vi "Write Tags.vi"(8 "error in (no error)":errorcluster, 11 "State in":T1={"State"=enum."Idle", "Start Time"=timestamp(0 s since 1904-01-01), "Configuration"={"Cycle Period"=0.0, "Ismatech"={"VISA resource name"="", "Simulated?"=FALSE, "Pump Number"=1.0, "Reverse?"=FALSE}, "Masterflex"={"VISA resource name"="", "Simulated?"=FALSE, "Pump Number"=1.0, "Reverse?"=FALSE}, "Mettler"={"VISA resource name"="", "Simulated?"=FALSE}, "Bronkhorst M13 Flow Meter"={"VISA resource name"="", "Simulated?"=FALSE, "Smoothing Steps"=1}, "PID 2 Parameters"={"Input Device"=enum."Bronkhorst M13", "Output Device"=enum."Ismatec ISM 831C", "Setpoint"=0.0, "PID gains"={"proportional gain (Kc)"=1.0, "integral time (Ti, min)"=0.01, "derivative time (Td, min)"=0.0}}, "Manual Entry"=0.0, "Auto?"=TRUE, "PID range"={"PID High"=100.0, "PID Low"=0.0, "High Warning"=100.0}, "Tacmina Settings"={"Analog DAQ Task"="", "Digital DAQ Task"=""}, "KNF SIMDOS Settings"={"VISA resource name"="", "Simulated?"=TRUE}, "ASIA Pump C"={"ASIA Pump #"=0, "channel"=0, "Simulated"=FALSE}, "VICI Settings"={"VISA resource name"="", "Pump ID"="", "Pump Head Vol"=0.0, "Reverse?"=FALSE, "Simulated?"=FALSE}, "FLOM Settings"={"VISA resource name"="", "Simulated?"=TRUE, "Pump Number"=0.0}, "SSI PR/LD Settings"={"VISA resource name"="", "Simulated?"=FALSE}, "Masterflex 75211 Settings"={"Analog DAQ Task"="", "Digital DAQ Task"=""}, "SSI P40 Settings"={"VISA resource name"="", "Simulated?"=TRUE}, "Ismatech 3 Channel Settings"={"VISA resource name"="", "Pump Number"=1, "Channel Number"=0, "Simulated?"=TRUE, "Reverse?"=FALSE}, "Bronkhorst M14 Settings"={"VISA resource name"="", "Simulated?"=FALSE, "Smoothing Steps"=1}, "Reset Totalizer"=FALSE, "Input Num Alarm Settings"=[], "Control Type"=enum."g/min", "Front End Display Options"={"Temperature"=TRUE, "Scale Grams"=FALSE, "Density"=TRUE, "Flow (g/min)"=FALSE, "Flow (ml/min)"=TRUE, "PSIG"=TRUE, "Total Grams"=TRUE, "Updated"=TRUE}}, "Current Time"=timestamp(0 s since 1904-01-01), "PID 1 Parameters"={"Setpoint"=0.0, "PID gains"={"proportional gain (Kc)"=1.0, "integral time (Ti, min)"=0.01, "derivative time (Td, min)"=0.0}}, "First Iteration"=FALSE, "Data"={"Flowmeter (g/min)"=0.0, "Flowmeter (ml/min)"=0.0, "Density"=0.0, "FL Temp"=0.0, "Scale Output (g)"=0.0, "Scale Rate of Change (g/min)"=0.0, "PID 1 Output"=0.0, "PID 2 Process Variable"=0.0, "PID 2 output"=0.0, "Pump Flow"=0.0, "Pump Pressure"=0.0, "Totalized Value"=0.0}, "Process Name"="", "Pump On?"=enum."Off", "Input Error"=FALSE, "Output Error"=FALSE, "Log Started"=FALSE, "PID Overshoot"=FALSE, "Current Setpoint"=0.0} {"PID 1 Parameters"."PID gains"."derivative time (Td, min)" format="%.3f"; "PID 1 Parameters"."PID gains"."integral time (Ti, min)" format="%.3f"; "PID 1 Parameters"."PID gains"."proportional gain (Kc)" format="%.3f"; "Configuration"."Bronkhorst M14 Settings"."Smoothing Steps" min=1 step=1; "Configuration"."Ismatech 3 Channel Settings"."Channel Number" min=0 max=3; "Configuration"."Ismatech 3 Channel Settings"."Pump Number" min=1; "Configuration"."PID range"."PID Low" min=0.0 max=100.0 format="%.2f"; "Configuration"."PID range"."PID High" format="%.2f"; "Configuration"."PID 2 Parameters"."PID gains"."derivative time (Td, min)" format="%.3f"; "Configuration"."PID 2 Parameters"."PID gains"."integral time (Ti, min)" format="%.3f"; "Configuration"."PID 2 Parameters"."PID gains"."proportional gain (Kc)" format="%.3f"; "Configuration"."Bronkhorst M13 Flow Meter"."Smoothing Steps" min=1 step=1; "Configuration"."ASIA Pump C"."channel" min=0 max=1 step=1; "Configuration"."Ismatech"."Pump Number" min=1.0 max=20.0 step=1.0; "Configuration"."Masterflex"."Pump Number" min=1.0 max=20.0 step=1.0}) -> (0 "error out":errorcluster, 3 "State out":T1={"State"=enum."Idle", "Start Time"=timestamp(0 s since 1904-01-01), "Configuration"={"Cycle Period"=0.0, "Ismatech"={"VISA resource name"="", "Simulated?"=FALSE, "Pump Number"=1.0, "Reverse?"=FALSE}, "Masterflex"={"VISA resource name"="", "Simulated?"=FALSE, "Pump Number"=1.0, "Reverse?"=FALSE}, "Mettler"={"VISA resource name"="", "Simulated?"=FALSE}, "Bronkhorst M13 Flow Meter"={"VISA resource name"="", "Simulated?"=FALSE, "Smoothing Steps"=1}, "PID 2 Parameters"={"Input Device"=enum."Bronkhorst M13", "Output Device"=enum."Ismatec ISM 831C", "Setpoint"=0.0, "PID gains"={"proportional gain (Kc)"=1.0, "integral time (Ti, min)"=0.01, "derivative time (Td, min)"=0.0}}, "Manual Entry"=0.0, "Auto?"=TRUE, "PID range"={"PID High"=100.0, "PID Low"=0.0, "High Warning"=100.0}, "Tacmina Settings"={"Analog DAQ Task"="", "Digital DAQ Task"=""}, "KNF SIMDOS Settings"={"VISA resource name"="", "Simulated?"=TRUE}, "ASIA Pump C"={"ASIA Pump #"=0, "channel"=0, "Simulated"=FALSE}, "VICI Settings"={"VISA resource name"="", "Pump ID"="", "Pump Head Vol"=0.0, "Reverse?"=FALSE, "Simulated?"=FALSE}, "FLOM Settings"={"VISA resource name"="", "Simulated?"=TRUE, "Pump Number"=0.0}, "SSI PR/LD Settings"={"VISA resource name"="", "Simulated?"=FALSE}, "Masterflex 75211 Settings"={"Analog DAQ Task"="", "Digital DAQ Task"=""}, "SSI P40 Settings"={"VISA resource name"="", "Simulated?"=TRUE}, "Ismatech 3 Channel Settings"={"VISA resource name"="", "Pump Number"=1, "Channel Number"=0, "Simulated?"=TRUE, "Reverse?"=FALSE}, "Bronkhorst M14 Settings"={"VISA resource name"="", "Simulated?"=FALSE, "Smoothing Steps"=1}, "Reset Totalizer"=FALSE, "Input Num Alarm Settings"=[], "Control Type"=enum."g/min", "Front End Display Options"={"Temperature"=TRUE, "Scale Grams"=FALSE, "Density"=TRUE, "Flow (g/min)"=FALSE, "Flow (ml/min)"=TRUE, "PSIG"=TRUE, "Total Grams"=TRUE, "Updated"=TRUE}}, "Current Time"=timestamp(0 s since 1904-01-01), "PID 1 Parameters"={"Setpoint"=0.0, "PID gains"={"proportional gain (Kc)"=1.0, "integral time (Ti, min)"=0.01, "derivative time (Td, min)"=0.0}}, "First Iteration"=FALSE, "Data"={"Flowmeter (g/min)"=0.0, "Flowmeter (ml/min)"=0.0, "Density"=0.0, "FL Temp"=0.0, "Scale Output (g)"=0.0, "Scale Rate of Change (g/min)"=0.0, "PID 1 Output"=0.0, "PID 2 Process Variable"=0.0, "PID 2 output"=0.0, "Pump Flow"=0.0, "Pump Pressure"=0.0, "Totalized Value"=0.0}, "Process Name"="", "Pump On?"=enum."Off", "Input Error"=FALSE, "Output Error"=FALSE, "Log Started"=FALSE, "PID Overshoot"=FALSE, "Current Setpoint"=0.0} {"PID 1 Parameters"."PID gains"."derivative time (Td, min)" format="%.3f"; "PID 1 Parameters"."PID gains"."integral time (Ti, min)" format="%.3f"; "PID 1 Parameters"."PID gains"."proportional gain (Kc)" format="%.3f"; "Configuration"."Bronkhorst M14 Settings"."Smoothing Steps" min=1 step=1; "Configuration"."Ismatech 3 Channel Settings"."Channel Number" min=0 max=3; "Configuration"."Ismatech 3 Channel Settings"."Pump Number" min=1; "Configuration"."PID range"."PID Low" min=0.0 max=100.0 format="%.2f"; "Configuration"."PID range"."PID High" format="%.2f"; "Configuration"."PID 2 Parameters"."PID gains"."derivative time (Td, min)" format="%.3f"; "Configuration"."PID 2 Parameters"."PID gains"."integral time (Ti, min)" format="%.3f"; "Configuration"."PID 2 Parameters"."PID gains"."proportional gain (Kc)" format="%.3f"; "Configuration"."Bronkhorst M13 Flow Meter"."Smoothing Steps" min=1 step=1; "Configuration"."ASIA Pump C"."channel" min=0 max=1 step=1; "Configuration"."Ismatech"."Pump Number" min=1.0 max=20.0 step=1.0; "Configuration"."Masterflex"."Pump Number" min=1.0 max=20.0 step=1.0})   [LabVIEW 2018, in "Feed Module.lvlib" / "Feed Module Engine.lvlib"]
uses:
  Feed Module Engine.lvlib
  State Cluster.ctl
  State Enum.ctl
  Feed Module/Controls/Feed Module Settings Cluster.ctl
  Ismatec ISM 831C/Controls/Ismatech ISM831C Settings Cluster.ctl
  Masterflex 7550-30/Controls/Settings Cluster.ctl
  Mettler Toledo/Controls/Settings Cluster.ctl
  Bronkhorst M13 Flow Meter/Settings Cluster.ctl
  PID 2 Parameters Cluster.ctl
  PID Input Enum.ctl
  PID 2 Output Enum.ctl
  Tacmina QI/Tacmina QI DAQ Setting.ctl
  KNF Pump/Settings Cluster plus SIMDOS.ctl
  ASIA Pump/Pump Settings.ctl
  VICI M50 Party Mode/Settings Cluster.ctl
  FLOM Pump/Settings Cluster.ctl
  SSI PR Class/SSI PR or LD Settings Cluster.ctl
  Masterflex 75211/Masterflex 75211 DAQ Setting.ctl
  SSI PR Class/SSI P40 Settings Cluster.ctl
  Ismatec 78001/Ismatec 4083.ctl
  Bronkhorst M14 Flow Meter/Settings Cluster.ctl
  Tag VIs/Numeric Alarm Settings Cluster.ctl
  PID 1 Parameters Cluster.ctl
  Tag VIs/Tag FGV Operation Enum.ctl
  Shared Variables/Dynamic Shared Variables.lvlib
  Feed Module/Feed Module.lvlib
  Ismatec ISM 831C/Ismatec ISM 831C.lvlib
  Masterflex 7550-30/Masterflex 7550-30.lvlib
  Mettler Toledo/Mettler Toledo.lvlib
  Bronkhorst M13 Flow Meter/Bronkhorst M13 Flow Meter.lvlib
  Tacmina QI/Tacmina QI.lvlib
  KNF Pump/KNF SIMDOS.lvlib
  ASIA Pump.lvlib
  VICI M50 Party Mode/VICI M6 M50 Party Mode.lvlib
  FLOM Pump/FLOM Pump.lvlib
  SSI PR Class/SSI PR or LD Pump.lvlib
  Masterflex 75211/Masterflex 75211.lvlib
  SSI PR Class/SSI P40 Pump.lvlib
  Ismatec 78001/Ismatec 4308.lvlib
  Bronkhorst M14 Flow Meter/Bronkhorst M14 Flow Meter.lvlib
panel:
  # "Output Instruments"
  # "Input Instruments"
  # "Output Instruments"
  # "Input Instruments"
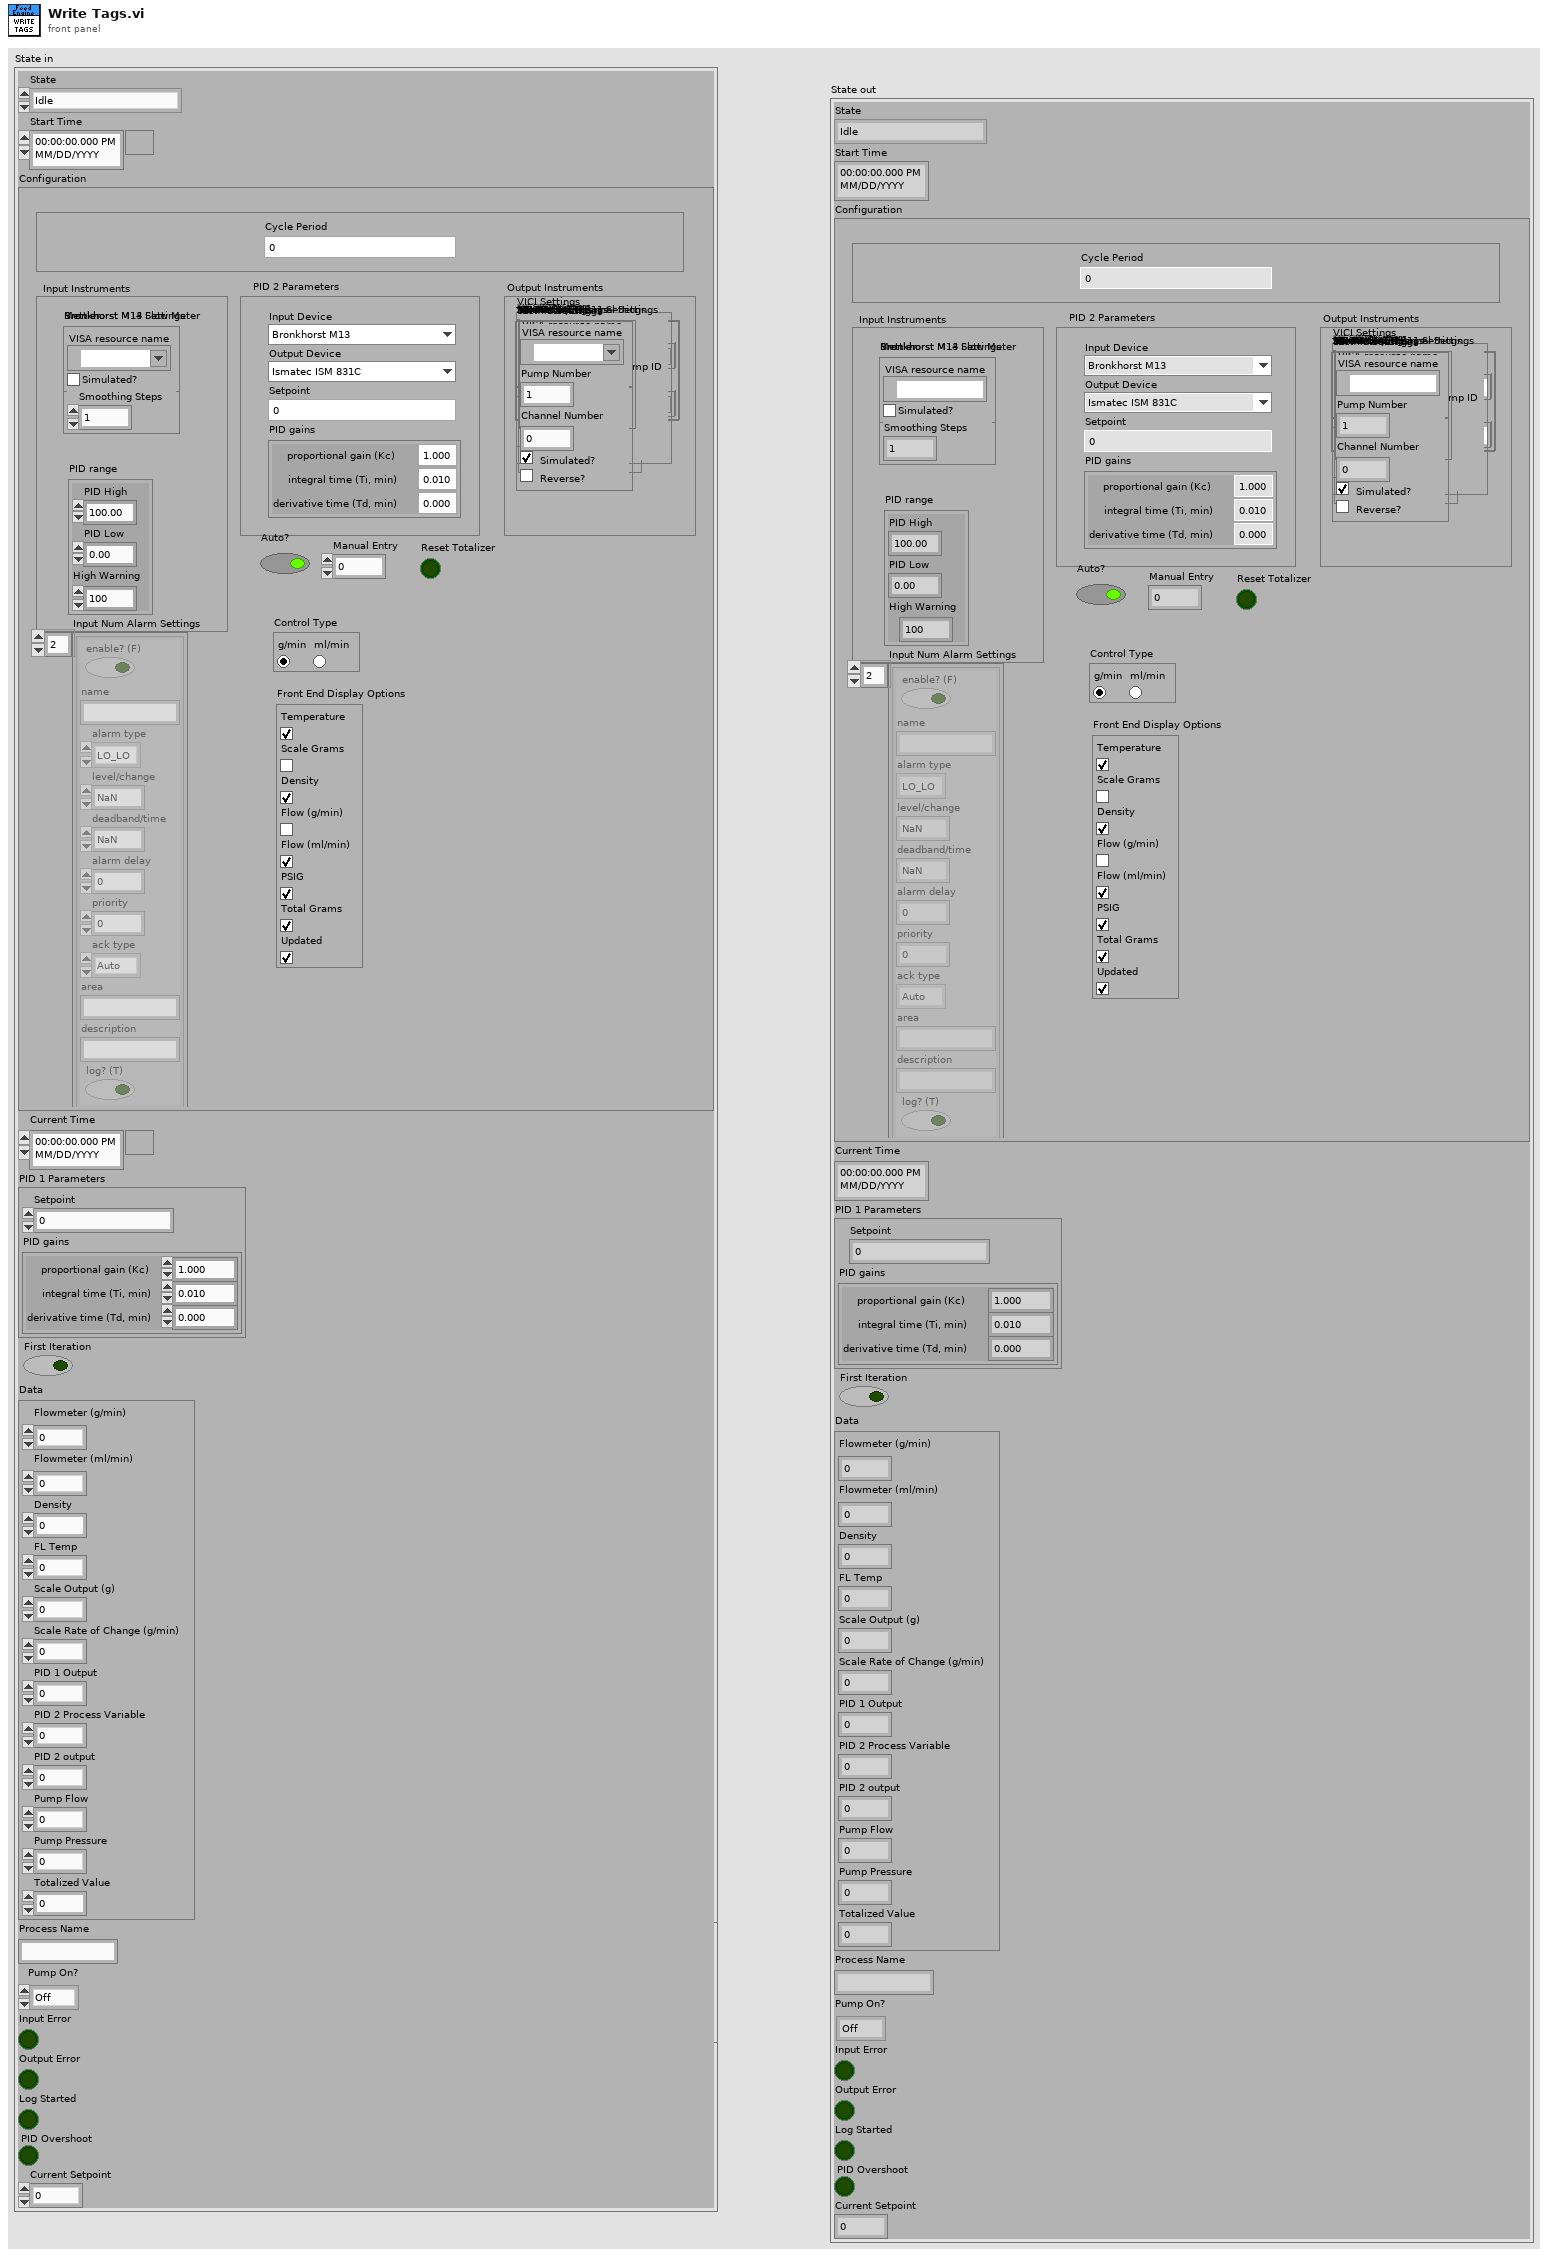
[diagram p1: front panel]
types:
  T1 = typedef "Feed Module.lvlib/Feed Module Engine.lvlib/State Cluster.ctl" = cluster{"State":T2, "Start Time":timestamp, "Configuration":T3, "Current Time":timestamp, "PID 1 Parameters":T22, "First Iteration":bool, "Data":cluster{"Flowmeter (g/min)":dbl, "Flowmeter (ml/min)":dbl, "Density":dbl, "FL Temp":dbl, "Scale Output (g)":dbl, "Scale Rate of Change (g/min)":dbl, "PID 1 Output":dbl, "PID 2 Process Variable":dbl, "PID 2 output":dbl, "Pump Flow":dbl, "Pump Pressure":dbl, "Totalized Value":dbl}, "Process Name":string, "Pump On?":enum16{"Off", "On", "Not Initialized"}, "Input Error":bool, "Output Error":bool, "Log Started":bool, "PID Overshoot":bool, "Current Setpoint":dbl}
  T2 = typedef "Feed Module.lvlib/Feed Module Engine.lvlib/State Enum.ctl" = enum16{"Measuring", "Idle", "Paused"}
  T3 = typedef "Feed Module.lvlib/Feed Module Settings Cluster.ctl" = cluster{"Cycle Period":dbl, "Ismatech":T4, "Masterflex":T5, "Mettler":T6, "Bronkhorst M13 Flow Meter":T7, "PID 2 Parameters":T8, "Manual Entry":dbl, "Auto?":bool, "PID range":cluster{"PID High":dbl, "PID Low":dbl, "High Warning":dbl}, "Tacmina Settings":T11, "KNF SIMDOS Settings":T12, "ASIA Pump C":T13, "VICI Settings":T14, "FLOM Settings":T15, "SSI PR/LD Settings":T16, "Masterflex 75211 Settings":T17, "SSI P40 Settings":T18, "Ismatech 3 Channel Settings":T19, "Bronkhorst M14 Settings":T20, "Reset Totalizer":bool, "Input Num Alarm Settings":T21[], "Control Type":enum32{"g/min", "ml/min"}, "Front End Display Options":cluster{"Temperature":bool, "Scale Grams":bool, "Density":bool, "Flow (g/min)":bool, "Flow (ml/min)":bool, "PSIG":bool, "Total Grams":bool, "Updated":bool}}
  T4 = typedef "Ismatec ISM 831C.lvlib/Ismatech ISM831C Settings Cluster.ctl" = cluster{"VISA resource name":refnum<visa-resource-name>, "Simulated?":bool, "Pump Number":dbl, "Reverse?":bool}
  T5 = typedef "Masterflex 7550-30.lvlib/Settings Cluster.ctl" = cluster{"VISA resource name":refnum<visa-resource-name>, "Simulated?":bool, "Pump Number":dbl, "Reverse?":bool}
  T6 = typedef "Mettler Toledo.lvlib/Settings Cluster.ctl" = cluster{"VISA resource name":refnum<visa-resource-name>, "Simulated?":bool}
  T7 = typedef "Bronkhorst M13 Flow Meter.lvlib/Settings Cluster.ctl" = cluster{"VISA resource name":refnum<visa-resource-name>, "Simulated?":bool, "Smoothing Steps":i32}
  T8 = typedef "PID 2 Parameters Cluster.ctl" = cluster{"Input Device":T9, "Output Device":T10, "Setpoint":dbl, "PID gains":cluster{"proportional gain (Kc)":dbl, "integral time (Ti, min)":dbl, "derivative time (Td, min)":dbl}}
  T9 = typedef "PID Input Enum.ctl" = enum16{"Default", "Bronkhorst M13", "Bronkhorst M14", "Scale Rate of Change"}
  T10 = typedef "PID 2 Output Enum.ctl" = enum16{"Default", "Ismatec ISM 4308", "Ismatec ISM 831C", "Masterflex 7550-30", "VICI M6", "VICI M50", "Tacmina QI", "KNF SIMDOS", "ASIA Type C", "FLOM UI-22-11", "SSI PR/LD", "SSI P40", "Masterflex 75211-70"}
  T11 = typedef "Tacmina QI.lvlib/Tacmina QI DAQ Setting.ctl" = cluster{"Analog DAQ Task":refnum<k21>, "Digital DAQ Task":refnum<k21>}
  T12 = typedef "KNF SIMDOS.lvlib/Settings Cluster plus SIMDOS.ctl" = cluster{"VISA resource name":refnum<visa-resource-name>, "Simulated?":bool}
  T13 = typedef "ASIA Pump.lvlib/Pump Settings.ctl" = cluster{"ASIA Pump #":i32, "channel":i32, "Simulated":bool}
  T14 = typedef "VICI M6 M50 Party Mode.lvlib/Settings Cluster.ctl" = cluster{"VISA resource name":refnum<visa-resource-name>, "Pump ID":string, "Pump Head Vol":dbl, "Reverse?":bool, "Simulated?":bool}
  T15 = typedef "FLOM Pump.lvlib/Settings Cluster.ctl" = cluster{"VISA resource name":refnum<visa-resource-name>, "Simulated?":bool, "Pump Number":dbl}
  T16 = typedef "SSI PR or LD Pump.lvlib/SSI PR or LD Settings Cluster.ctl" = cluster{"VISA resource name":refnum<visa-resource-name>, "Simulated?":bool}
  T17 = typedef "Masterflex 75211.lvlib/Masterflex 75211 DAQ Setting.ctl" = cluster{"Analog DAQ Task":refnum<k21>, "Digital DAQ Task":refnum<k21>}
  T18 = typedef "SSI P40 Pump.lvlib/SSI P40 Settings Cluster.ctl" = cluster{"VISA resource name":refnum<visa-resource-name>, "Simulated?":bool}
  T19 = typedef "Ismatec 4308.lvlib/Ismatec 4083.ctl" = cluster{"VISA resource name":refnum<visa-resource-name>, "Pump Number":i16, "Channel Number":i16, "Simulated?":bool, "Reverse?":bool}
  T20 = typedef "Bronkhorst M14 Flow Meter.lvlib/Settings Cluster.ctl" = cluster{"VISA resource name":refnum<visa-resource-name>, "Simulated?":bool, "Smoothing Steps":i32}
  T21 = typedef "Numeric Alarm Settings Cluster.ctl" = cluster{"enable? (F)":bool, "name":string, "alarm type":enum16{"HI_HI", "HI", "LO", "LO_LO"}, "level/change":dbl, "deadband/time":dbl, "alarm delay":dbl, "priority":u32, "ack type":enum16{"Auto", "User", "None", "Each Occurrence"}, "area":string, "description":string, "log? (T)":bool}
  T22 = typedef "PID 1 Parameters Cluster.ctl" = cluster{"Setpoint":dbl, "PID gains":cluster{"proportional gain (Kc)":dbl, "integral time (Ti, min)":dbl, "derivative time (Td, min)":dbl}}
  T23 = typedef "Tag FGV Operation Enum.ctl" = enum16{"Init", "Set Notification Queue", "Create Tag", "Commit", "Write Tag (Numeric)", "Write Tag (Boolean)", "Read All Tags", "Read One Tag", "Delete Tag Category", "Set Alarm Parameters (Numeric)", "Set Alarm Parameters (Boolean)", "Enable All Alarms", "Disable All Alarms", "Delete All Tags", "Read Alarms", "Ack Alarm", "Read Alarm Parameters (Numeric)", "Read Alarm Parameters (Boolean)"}
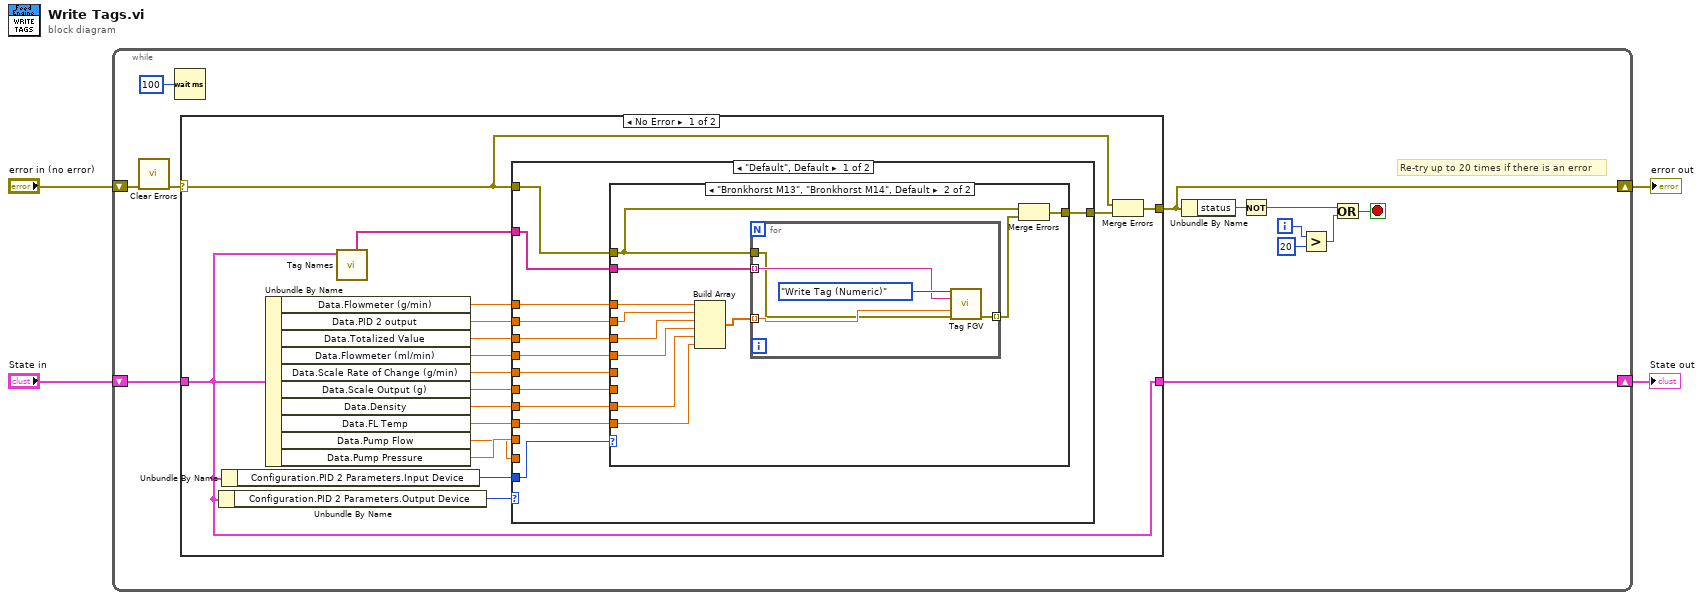
[diagram p0: block diagram]
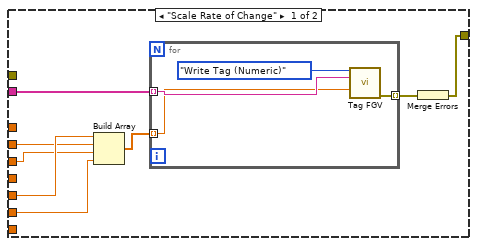
[diagram p2: hidden frame]
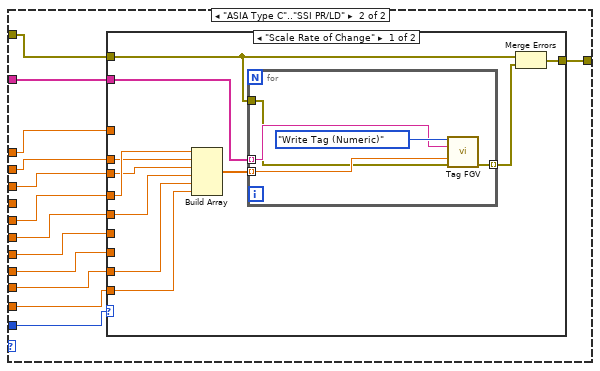
[diagram p3: hidden frame]
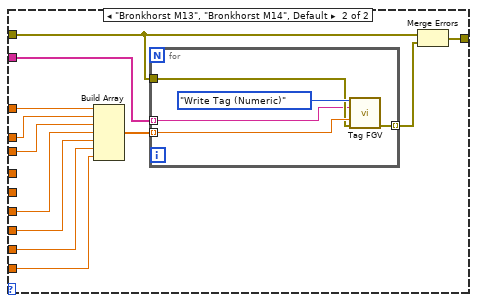
[diagram p4: hidden frame]
diagram:
  n1 = while {
    shift-right: [w10] -> w4
    shift-left: "error in (no error)" -> [w8]
    shift-right: [w15] -> w1
    shift-left: "State in" -> [w16]
    i -> [w6]
    stop <- w14 stop-if-true
    # "Re-try up to 20 times if there is an error"
    n2 = call <vilib>:"Clear Errors.vi"("error in (no error)"=w8) -> ("error out"=w7:errorcluster)  [unwired: 5 in, 1 out]
    n3 = Wait (ms)(milliseconds to wait=u32 100) -> ()  [unwired: 1 out]
    n4 = case shown="No Error" w7 {
      selector: w7 -> [w19 w121]
      tunnel: [w21 w121] -> w10
      tunnel: w16 -> [w26 w120]
      tunnel: [w26 w120] -> w15
      frame No Error {
        n5 = Unbundle By Name(w26) -> ("Configuration.PID 2 Parameters.Output Device"=w24:T10)
        n6 = Unbundle By Name(w26) -> ("Configuration.PID 2 Parameters.Input Device"=w33:T9)
        n7 = Unbundle By Name(w26) -> ("Data.Flowmeter (g/min)"=w29:dbl, "Data.PID 2 output"=w31:dbl, "Data.Totalized Value"=w18:dbl, "Data.Flowmeter (ml/min)"=w17:dbl, "Data.Scale Rate of Change (g/min)"=w32:dbl, "Data.Scale Output (g)"=w30:dbl, "Data.Density"=w28:dbl, "Data.FL Temp"=w27:dbl, "Data.Pump Flow"=w22:dbl, "Data.Pump Pressure"=w23:dbl)
        n8 = call "Tag Names.vi"("State in"=w26) -> ("All  Numeric Tags"=w25:string[])  [unwired: 6 in, 4 out]
        n9 = case shown="\"Default\", Default" w24 {
          tunnel: w33 -> [w36 w86]
          tunnel: w32 -> [w38 w85]
          tunnel: w31 -> [w41 w84]
          tunnel: w30 -> [w37 w83]
          tunnel: w29 -> [w42 w82]
          tunnel: w28 -> [w40 w81]
          tunnel: w27 -> [w39 w80]
          tunnel: w19 -> [w44 w79]
          tunnel: [w45 w78] -> w20
          tunnel: w25 -> [w43 w77]
          tunnel: w23 -> [_ w76]
          tunnel: w22 -> [_ w75]
          tunnel: w18 -> [w35 w74]
          tunnel: w17 -> [w34 _]
          frame "Default", Default {
            n10 = case shown="\"Bronkhorst M13\", \"Bronkhorst M14\", Default" w36 {
              tunnel: w43 -> [w53 w66]
              tunnel: w42 -> [_ w67]
              tunnel: [w47 w60] -> w45
              tunnel: w44 -> [_ w61]
              tunnel: w41 -> [w50 w65]
              tunnel: w40 -> [_ w64]
              tunnel: w39 -> [_ w63]
              tunnel: w38 -> [w51 _]
              tunnel: w37 -> [w49 _]
              tunnel: w35 -> [w46 w59]
              tunnel: w34 -> [_ w58]
              frame "Scale Rate of Change" {
                n11 = Build Array(w51, w50, w46, w49) -> (w52:dbl[])
                n12 = for {
                  tunnel: w53 -> [w56] mode=indexing
                  tunnel: w52 -> [w55] mode=indexing
                  tunnel: [w54] -> w48 mode=indexing
                  n13 = call "Tag FGV.vi"("Operation"=Tag_FGV_Operation_Enum."Write Tag (Numeric)", "Tag Name"=w56, "Data"=w55) -> ("error out"=w54:errorcluster)  [unwired: 5 in, 7 out]
                }
                n14 = Merge Errors(w48) -> (w47:errorcluster)
              }
              frame "Bronkhorst M13", "Bronkhorst M14", Default {
                n15 = Build Array(w67, w65, w59, w58, w64, w63) -> (w68:dbl[])
                n16 = for {
                  tunnel: w68 -> [w72] mode=indexing
                  tunnel: [w69] -> w62 mode=indexing
                  tunnel: w66 -> [w71] mode=indexing
                  tunnel: w61 -> [w70]
                  n17 = call "Tag FGV.vi"("Operation"=Tag_FGV_Operation_Enum."Write Tag (Numeric)", "Tag Name"=w71, "Data"=w72, "error in (no error)"=w70) -> ("error out"=w69:errorcluster)  [unwired: 4 in, 7 out]
                }
                n18 = Merge Errors(w61, w62) -> (w60:errorcluster)
              }
            }
          }
          frame "ASIA Type C".."SSI PR/LD" {
            n19 = case shown="\"Scale Rate of Change\"" w86 {
              tunnel: w77 -> [w97 w109]
              tunnel: w85 -> [w96 _]
              tunnel: w84 -> [w95 w114]
              tunnel: w83 -> [w94 _]
              tunnel: w82 -> [_ w112]
              tunnel: w81 -> [_ w111]
              tunnel: w80 -> [_ w110]
              tunnel: w79 -> [w89 w105]
              tunnel: [w88 w104] -> w78
              tunnel: w76 -> [w92 w108]
              tunnel: w75 -> [w91 w107]
              tunnel: w74 -> [w87 w103]
              frame "Scale Rate of Change" {
                n20 = Build Array(w96, w95, w87, w94, w92, w91) -> (w93:dbl[])
                n21 = for {
                  tunnel: w97 -> [w101] mode=indexing
                  tunnel: w93 -> [w100] mode=indexing
                  tunnel: w89 -> [w99]
                  tunnel: [w98] -> w90 mode=indexing
                  n22 = call "Tag FGV.vi"("Operation"=Tag_FGV_Operation_Enum."Write Tag (Numeric)", "Tag Name"=w101, "Data"=w100, "error in (no error)"=w99) -> ("error out"=w98:errorcluster)  [unwired: 4 in, 7 out]
                }
                n23 = Merge Errors(w89, w90) -> (w88:errorcluster)
              }
              frame "Bronkhorst M13", "Bronkhorst M14", Default {
                n24 = Build Array(w112, w114, w103, w111, w110, w108, w107) -> (w113:dbl[])
                n25 = for {
                  tunnel: w113 -> [w118] mode=indexing
                  tunnel: w105 -> [w117]
                  tunnel: [w116] -> w106 mode=indexing
                  tunnel: w109 -> [w115] mode=indexing
                  n26 = call "Tag FGV.vi"("Operation"=Tag_FGV_Operation_Enum."Write Tag (Numeric)", "Tag Name"=w115, "Data"=w118, "error in (no error)"=w117) -> ("error out"=w116:errorcluster)  [unwired: 4 in, 7 out]
                }
                n27 = Merge Errors(w105, w106) -> (w104:errorcluster)
              }
            }
          }
        }
        n28 = Merge Errors(w19, w20) -> (w21:errorcluster)
      }
      frame Error {
      }
    }
    n29 = Unbundle By Name(w10) -> ("status"=w9:bool)
    n30 = Not(x=w9) -> (.not. x?=w13:bool)
    n31 = Greater?(x=w6, y=20) -> (0:w11:bool)
    n32 = Or(x=w13, y=w11) -> (x .or. y?=w14:bool)
  }
  "error out" <- w4
  "State out" <- w1
